vi "Publish Data.vi"(8 "error in (no error)":errorcluster, 9 "Message Priority (Normal)":T1=enum."Normal", 10 "Data to Publish":refnum<class "Data.lvclass">, 11 "Actor in":refnum<class "Actor.lvclass">) -> (0 "error out":errorcluster, 1 "Dropped?":bool, 3 "Actor out":refnum<class "Actor.lvclass">)   [LabVIEW 2020, in "Publisher.lvlib" / "Publish Msg.lvclass"]
doc: "This VI sends the data to the Publisher for publishing."
uses:
  Publish Msg.lvclass
  PPL/HDH.Actor Framework.Core.Actor.lvlibp/1abvi3w/vi.lib/ActorFramework/Actor/Actor.lvclass
  PPL/HDH.Actor Framework.Core.Actor.lvlibp/1abvi3w/vi.lib/ActorFramework/Message Enqueuer/Message Priority.ctl
  PPL/HDH.Data.Generic.lvlibp/Data.lvclass
  Messages/Data Msg/Data Msg.lvclass/Data Msg.ctl
  Publish Msg.lvclass/Publish Msg.ctl
  Messages/Data Msg/Data Msg.lvclass
  C:/Current projects/WS/PPL/HDH.Actor Framework.Core.Actor.lvlibp/1abvi3w/vi.lib/ActorFramework/Message/Message.lvclass
  C:/Current projects/WS/Framework/Framework/Actors/Publisher/Publisher Messages/Publisher Msg/Publisher Msg.lvclass
  Publisher Msg/Send To Caller.vi
  PPL/HDH.Actor Framework.Core.Actor.lvlibp/1abvi3w/vi.lib/ActorFramework/Message Enqueuer/Message Enqueuer.lvclass
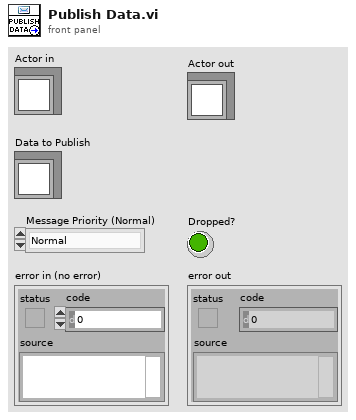
[diagram p1: front panel]
types:
  T1 = typedef "HDH.Actor Framework.Core.Actor.lvlibp/Message Enqueuer.lvclass/Message Priority.ctl" = enum16{"Low", "Normal", "High"}
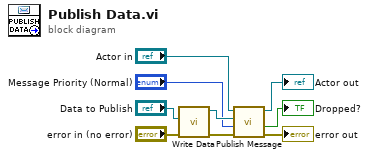
[diagram p0: block diagram]
diagram:
  n1 = call "Write Data.vi"("error in (no error)"="error in (no error)", "Data"="Data to Publish") -> ("error out"=w4:errorcluster, "Data Msg out"=w7:refnum<class "Data Msg.lvclass">)  [unwired: 8 in]
  n2 = call "Publish Message.vi"("error in (no error)"=w4, "Message Priority (Normal)"="Message Priority (Normal)", "Message to Publish"=w7, "Actor in"="Actor in") -> ("error out"=→"error out":errorcluster, "Dropped?"=→"Dropped?":bool, "Actor out"=→"Actor out":refnum<class "Actor.lvclass">)  [unwired: 5 in]
